vi "Host main.vi"() -> ()   [LabVIEW 2018]
panel:
  in  "Minimize":bool
  in  "Close":bool
  in  "Config":bool
  in  "Start":bool
  out "Nível dos tanques":dbl(graph) caption="Waveform Chart"
  out "Tensão nas Bombas":dbl(graph) caption="Waveform Chart"
  in  "Valvula proporcional 2":dbl=7.5
  in  "Valvula proporcional 1":dbl=7.5
  out "Tanque 4":T1 scale=0.0..20.0
  out "Tanque 3":T1 scale=0.0..20.0
  out "Tanque 2":T1 scale=0.0..20.0
  out "Tanque 1":T1 scale=0.0..20.0
  in  "Valvula 4":bool
  in  "Valvula 3":bool
  in  "Valvula 1":bool
  in  "Valvula 2":bool
  in  "Pump 2":dbl=3.0 min=0.0 format="%.2f"
  in  "Pump 1":dbl=3.0 min=0.0 format="%.2f"
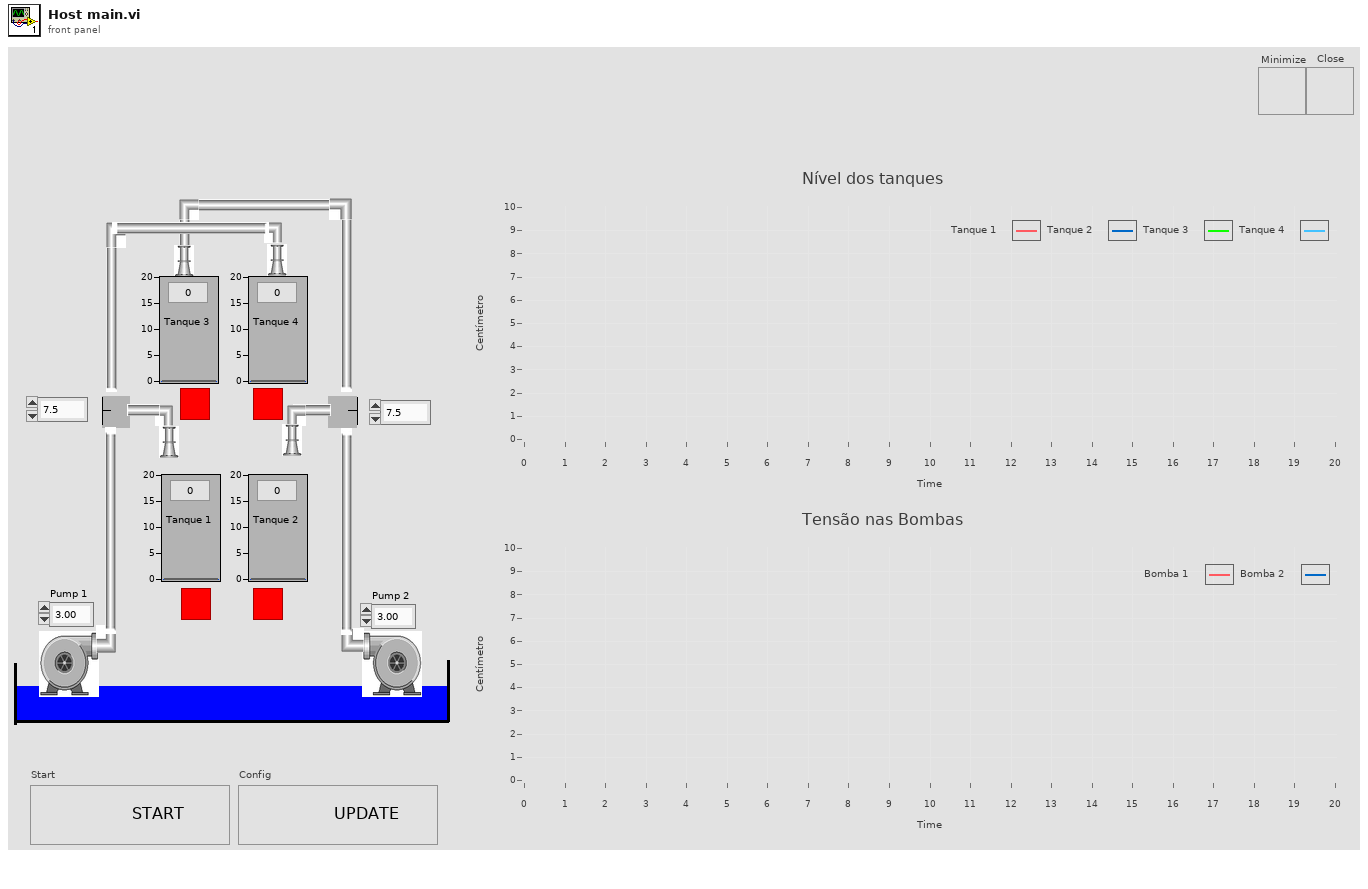
[diagram p1: front panel]
types:
  T1 = typedef "Tanque.ctl" = dbl
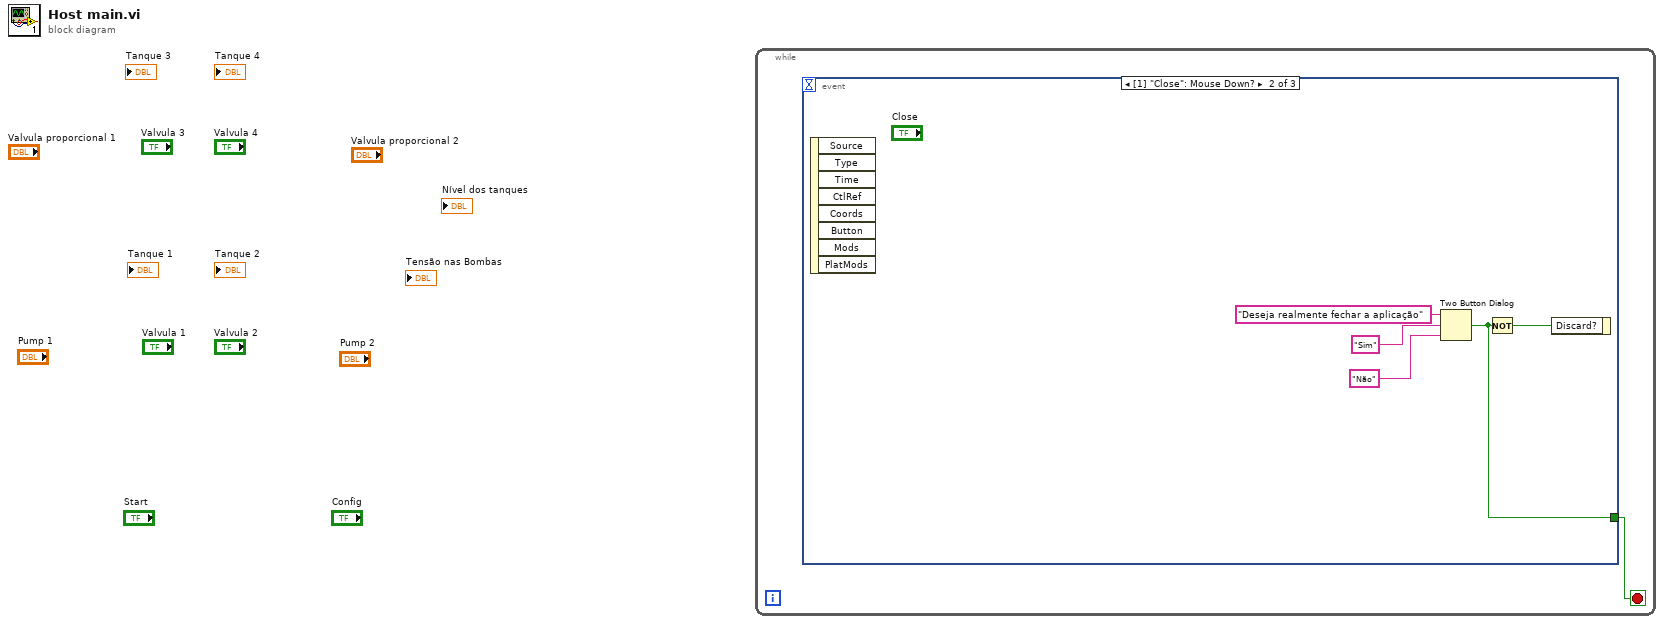
[diagram p0: block diagram]
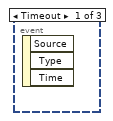
[diagram p2: hidden frame]
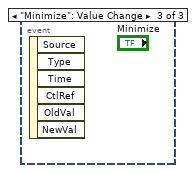
[diagram p3: hidden frame]
diagram:
  n1 = while {
    stop <- w1 stop-if-true
    n2 = event shown="[1] \"Close\": Mouse Down?" {
      selector: _ -> [_ _ _]
      dyn-events: _ -> [_ _ _]
      timeout: _ -> [_ _ _]
      tunnel: [_ w2 _] -> w1
      event Timeout {
        n3 = event-data() -> ()  [unwired: 1 in, 3 out]
      }
      event "Close": Mouse Down? {
        n4 = event-data() -> ()  [unwired: 1 in, 8 out]
        n5 = Two Button Dialog(message="Deseja realmente fechar a aplicação", 1:"Não" ("F button name (\"Cancel\")"), 2:"Sim" ("T button name (\"OK\")")) -> (T button?=w2:bool)
        n6 = Not(x=w2) -> (.not. x?=w6:bool)
        n7 = event-data("Discard?"=w6) -> ()  [unwired: 1 in, 1 out]
      }
      event "Minimize": Value Change {
        n8 = event-data() -> ()  [unwired: 1 in, 6 out]
      }
    }
  }
